vi "Host Approach Retraction.vi"() -> ()   [LabVIEW 2013]
uses:
  <vilib>/rvi/interface/nirviOpenFPGA/nirviOpenFPGA.xnode
  <vilib>/rvi/interface/nirviReadWriteControl/nirviReadWriteControl.xnode
  <vilib>/rvi/interface/nirviCloseFPGA/nirviCloseFPGA.xnode
  <vilib>/FPGAPlugInAG/Dynamic/niLvFpga_Close_Dynamic.vi
  <vilib>/rvi/interface/Simulation/niFpgaSimulationCallBeginRW.vi
  <vilib>/rvi/errors/niLvFpgaAdjustHostInterfaceError.vi
  <vilib>/rvi/interface/nirviMethod/nirviMethod.xnode
  <vilib>/FPGAPlugInAG/Dynamic/niLvFpga_Run_Dynamic.vi
panel:
  out "FPGA Output Voltage":dbl(graph)
  in  "MCL Counter":i64
  in  "MCL Divisions":i32
  out "MCL Range Indicator":bool
  out "Host Counter Indicator":i64
  out "Digital Steps per Region":i32
  out "Host Counter Output":i32
  in  "Z Position MCL Fine":i32
  out "Host Z Position Indicator":i32
  out "Z Position Range Indicator":bool
  out "Z Fine Steps per Region":dbl
  out "Host Z Output":fxp<+/-,40,30>
  in  "Manual Approach Start":bool
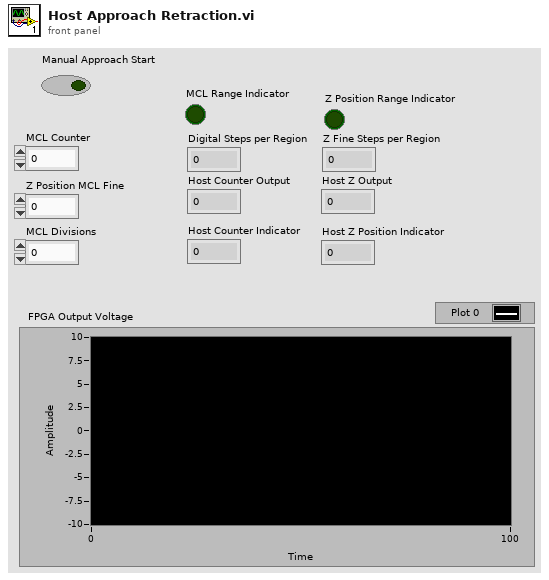
[diagram p1: front panel]
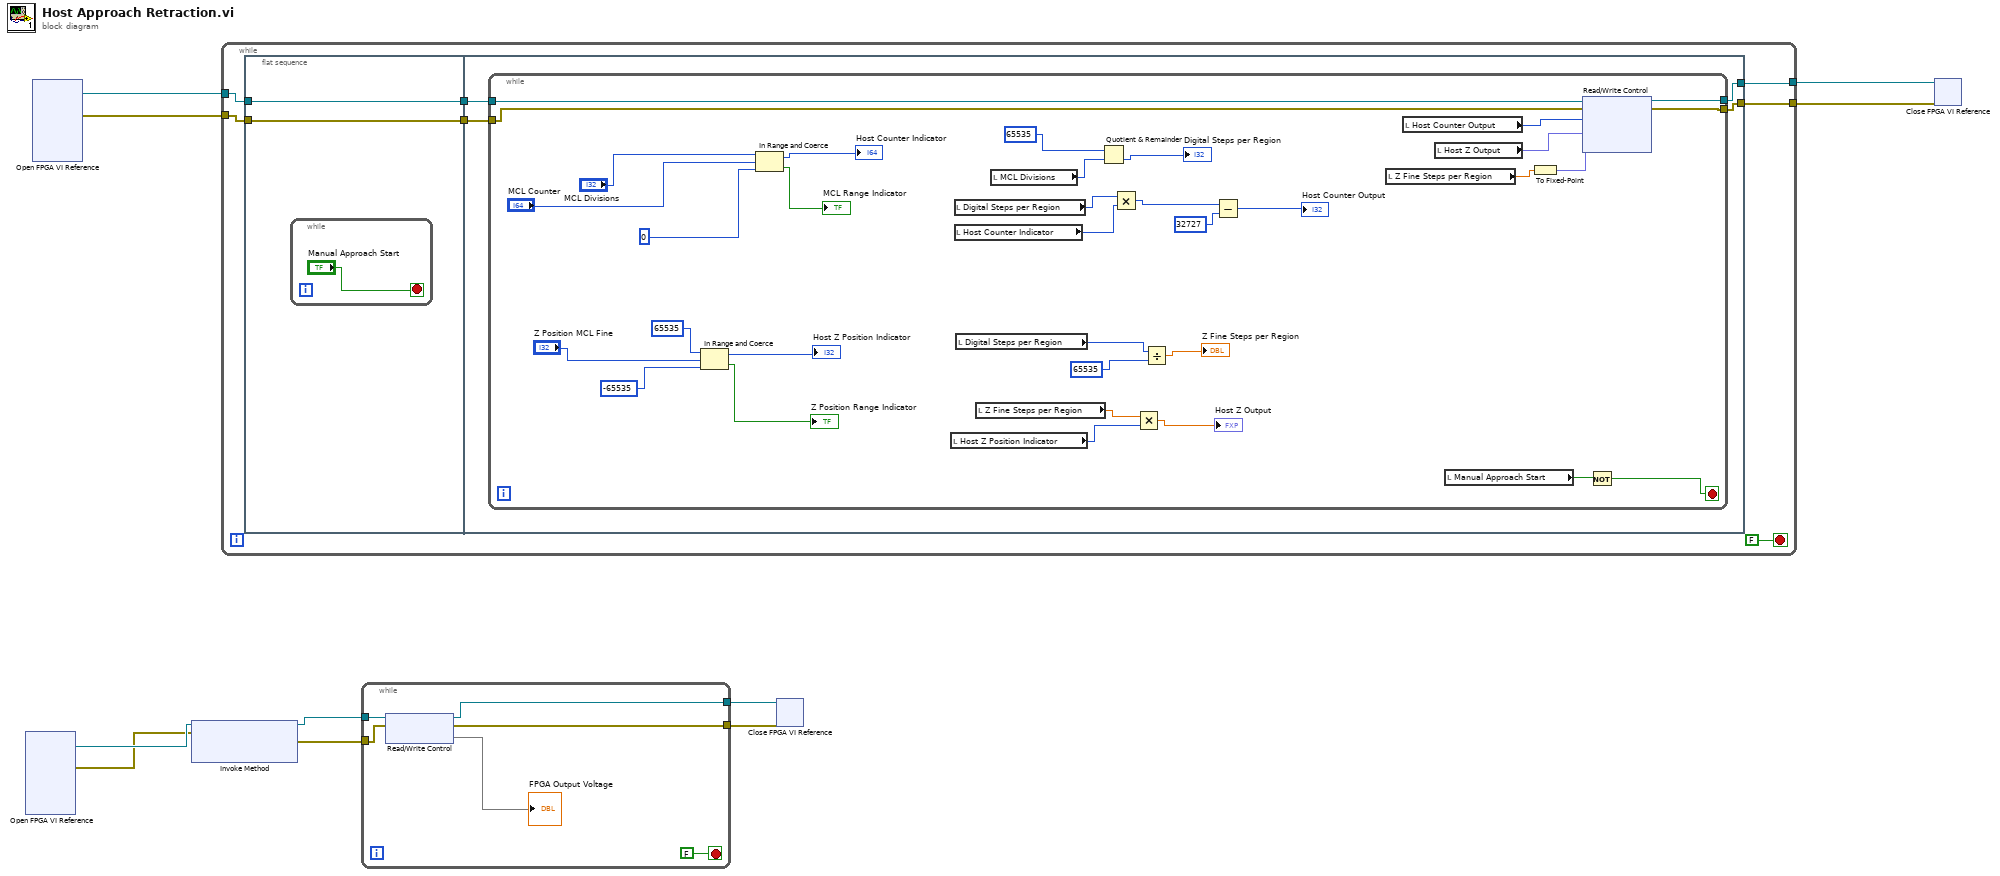
[diagram p0: block diagram]
diagram:
  n1 = xnode "Open FPGA VI Reference"() -> ("FPGA VI Reference Out"=w2:refnum<k20>, "error out"=w1:errorcluster)  [unwired: 2 in]
  n2 = xnode "Open FPGA VI Reference"() -> ("FPGA VI Reference Out"=w8:refnum<k20>, "error out"=w7:errorcluster)  [unwired: 2 in]
  n3 = xnode "Invoke Method"("FPGA VI Reference In"=w2, "error in"=w1) -> ("FPGA VI Reference Out"=w4:refnum<k20>, "error out"=w3:errorcluster)  [unwired: 1 in]
  n4 = while {
    tunnel: [w16] -> w10
    tunnel: [w15] -> w9
    tunnel: w8 -> [w13]
    tunnel: w7 -> [w11]
    stop <- FALSE stop-if-true
    n5 = flat-sequence {
      tunnel: [w19] -> w14
      tunnel: w13 -> [w19]
      tunnel: [w18] -> w12
      tunnel: w11 -> [w18]
      tunnel: [w22] -> w16
      tunnel: [w21] -> w15
      tunnel: w14 -> [w24]
      tunnel: w12 -> [w23]
      frame #0 {
        n6 = while {
          stop <- "Manual Approach Start" stop-if-true
        }
      }
      frame #1 {
        n7 = while {
          tunnel: w24 -> [w58]
          tunnel: w23 -> [w57]
          tunnel: [w56] -> w22
          tunnel: [w55] -> w21
          stop <- w53 stop-if-true
          n8 = In Range and Coerce(upper limit=65535, x="Z Position MCL Fine", lower limit=-65535) -> (coerced(x)=→"Host Z Position Indicator":i32, In Range?=→"Z Position Range Indicator":bool)
          n9 = In Range and Coerce(upper limit="MCL Divisions", x="MCL Counter", lower limit=0) -> (coerced(x)=→"Host Counter Indicator":i64, In Range?=→"MCL Range Indicator":bool)
          n10 = local read "Host Z Position Indicator"() -> (w29:i32)
          n11 = local read "Digital Steps per Region"() -> (w42:i32)
          n12 = local read "Host Counter Indicator"() -> (w41:i64)
          n13 = local read "Digital Steps per Region"() -> (w33:i32)
          n14 = local read "Z Fine Steps per Region"() -> (w30:dbl)
          n15 = local read "MCL Divisions"() -> (w46:i32)
          n16 = Quotient & Remainder(x=65535, y=w46) -> (floor(x/y)=→"Digital Steps per Region":i32)  [unwired: 1 out]
          n17 = Multiply(x=w42, y=w41) -> (x*y=w43:i64)
          n18 = Multiply(x=w30, y=w29) -> (x*y=→"Host Z Output":dbl)
          n19 = Divide(x=w33, y=65535) -> (x/y=→"Z Fine Steps per Region":dbl)
          n20 = Subtract(x=w43, y=32727) -> (x-y=→"Host Counter Output":i64)
          n21 = local read "Z Fine Steps per Region"() -> (w25:dbl)
          n22 = local read "Host Counter Output"() -> (w39:i32)
          n23 = local read "Host Z Output"() -> (w27:fxp<+/-,40,30>)
          n24 = local read "Manual Approach Start"() -> (w54:bool)
          n25 = To Fixed-Point(number=w25) -> (fixed-point=w26:fxp<+/-,32,16>)  [unwired: 1 in]
          n26 = xnode "Read/Write Control"("FPGA VI Reference In"=w58, "error in"=w57, "Unselected"=w39, "Unselected"=w27, "Unselected"=w26) -> ("FPGA VI Reference Out"=w56:refnum<k20>, "error out"=w55:errorcluster)
          n27 = Not(x=w54) -> (.not. x?=w53:bool)
        }
      }
    }
  }
  n28 = while {
    tunnel: w4 -> [w63]
    tunnel: w3 -> [w62]
    tunnel: [w61] -> w6
    tunnel: [w60] -> w5
    stop <- FALSE stop-if-true
    n29 = xnode "Read/Write Control"("FPGA VI Reference In"=w63, "error in"=w62) -> ("FPGA VI Reference Out"=w61:refnum<k20>, "error out"=w60:errorcluster, "Unselected"=→"FPGA Output Voltage")
  }
  n30 = xnode "Close FPGA VI Reference"("FPGA VI Reference In"=w6, "error in"=w5) -> ()  [unwired: 1 out]
  n31 = xnode "Close FPGA VI Reference"("FPGA VI Reference In"=w10, "error in"=w9) -> ()  [unwired: 1 out]
